vi "Destroy User Events.vi"(11 "UI Template in":refnum<class "Database Provider.lvclass">) -> (3 "UI Template out":refnum<class "Database Provider.lvclass">)   [LabVIEW 2024, in "Database Provider.lvlib" / "Database Provider.lvclass"]
uses:
  Database Provider.lvclass
  Database Provider.lvclass/Database Provider.ctl
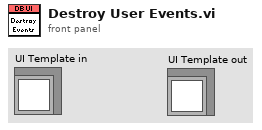
[diagram p1: front panel]
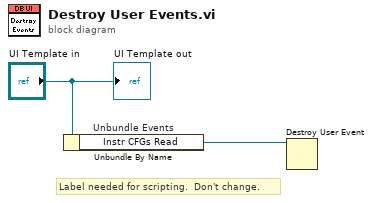
[diagram p0: block diagram]
diagram:
  # "Label needed for scripting.  Don't change."
  n1 = Unbundle By Name "Unbundle Events"("UI Template in") -> ("Instr CFGs Read"=w2:refnum<user-event>)
  n2 = Destroy User Event(user event=w2) -> ()  [unwired: 1 in, 1 out]
  "UI Template out" <- "UI Template in"
